vi "Set Inspection Type [FLM].vi"(7 "Micropulse # In":i32, 8 "error in (no error)":errorcluster, 10 "Inspection Type":T1) -> (0 "error out":errorcluster, 5 "Micropulse # Out":i32)   [LabVIEW 2026, in "MicroPulse_Driver.lvlib"]
doc: "Specifies the type of tests to be carried out at each inspection point. This can be conventional tests, phased array tests or both.\n\nFormat:\nFLM <Mode>\n\nDescription:\nInspections where MicroPulse is monitoring encoders and firing a test sequence on position it is necessary to determine the type of tests to be carried out at each inspection point.\n\nParameters:\n<mode> :\n0 = Performs convention tests only (CAL 0);\n1 = Performs convention tests and then Phased array tests (CAL 0 then CALS 0);\n2 = Performs Phased array tests and then Conventional tests (CALS 0 then CAL 0);\n3 = Performs Phased array tests only (CALS 0 );\n4 = Performs all enabled groups within the NUMG (CALG0);\n5 = Performs phased array sweep sequence as defined by the FDEF command. Alternatively perform a parallel Phased Array/Conventional test sequence if defined by the FDEF.\n\nExample:\nFLM 3 : Performs a CALS 0 on each inspection point"
uses:
  MicroPulse_Driver.lvlib
  Data/Datatypes/MP - fly inspection tests.ctl
  Private/MP-Registry Action-Enum.ctl
  <instrlib>/Micropulse/Micropulse.lvlib
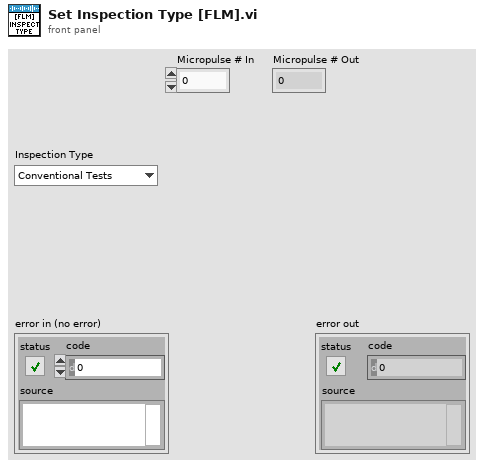
[diagram p1: front panel]
types:
  T1 = typedef "Micropulse.lvlib/MP - fly inspection tests.ctl" = enum16{"Conventional Tests", "Conv >> PA Tests", "PA >> Conv Tests", "PA Tests", "Group Tests", "PA Sweep as per FDEF"}
  T2 = typedef "MicroPulse_Driver.lvlib/MP-Registry Action-Enum.ctl" = enum16{"Read", "Add Test", "Add Command", "Add Gate Command", "Add Encoder Command", "Clear Command  List", "Set Registry", "Set System Details", "Set DOF", "Set Velocity", "Disable Asynch Reads", "Enable Asynch Reads", "Add Connection", "Disconnect", "Shutdown"}
  T3 = typedef "Micropulse.lvlib/TCP config.ctl" = cluster{"Connection ID":refnum<k5>, "IP address":string, "host port":u16, "OC timeout":i32, "Read timeout":i32, "Write timeout":i32}
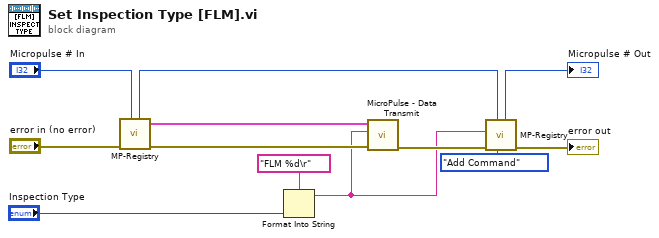
[diagram p0: block diagram]
diagram:
  n1 = call "MP-Registry.vi"("Micropulse # In"="Micropulse # In", "error in (no error)"="error in (no error)") -> ("error out"=w10:errorcluster, "TCP config"=w9:T3, "Micropulse # Out"=w6:i32)  [unwired: 6 in, 1 out]
  n2 = Format Into String(format string="FLM %d\r", "Inspection Type") -> (resulting string=w3:string)  [unwired: 2 in, 1 out]
  n3 = call "MicroPulse - Data Transmit.vi"("error in (no error)"=w10, "data"=w3, "TCP config"=w9) -> ("error out"=w7:errorcluster)  [unwired: 6 in, 2 out]
  n4 = call "MP-Registry.vi"("Action"=MP-Registry_Action-Enum."Add Command", "Micropulse # In"=w6, "error in (no error)"=w7, "Data in"=w3) -> ("error out"=→"error out":errorcluster, "Micropulse # Out"=→"Micropulse # Out":i32)  [unwired: 4 in, 2 out]
